vi "TF-Mini_LiDAR (SubVI).vi"(3 "UART Data":u16[](array[numeric])) -> (0 "Distance (cm)":dbl, 1 "Reading good?":bool)   [LabVIEW 2018]
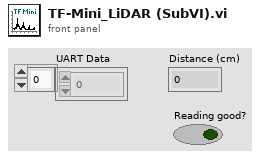
[diagram p1: front panel]
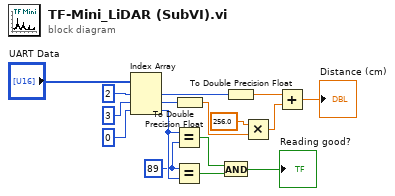
[diagram p0: block diagram]
diagram:
  w14 = u8 89 ("y")
  n1 = Index Array(array="UART Data", index #1=2 ("index"), index #2=3 ("index"), index #3=0 ("index")) -> (element #1=w5:u16, element #2=w4:u16, element #3=w15:u16)
  n2 = Equal?(x=w15, y=w14) -> (x = y?=w11:bool)
  n3 = Equal?(x=w14, y=w15) -> (x = y?=w12:bool)
  n4 = To Double Precision Float(number=w4) -> (double precision float=w6:dbl)
  n5 = And(x=w11, y=w12) -> (x .and. y?=→"Reading good?":bool)
  n6 = To Double Precision Float(number=w5) -> (double precision float=w9:dbl)
  n7 = Multiply(x=256.0, y=w6) -> (x*y=w8:dbl)
  n8 = Add(x=w9, y=w8) -> (x+y=→"Distance (cm)":dbl)
